vi "Get Or Create Cal Standard.vi"(11 "error in (no error)":errorcluster) -> (4 "Cal Standard Base out":refnum<class "Cal Standard Base.lvclass">, 15 "error out":errorcluster)   [LabVIEW 2023, in "RFFixtureCharact.Instruments.lvlib" / "Cal Standard Factory.lvclass"]
uses:
  Cal Standard Factory.lvclass
  Cal Standard Base/Cal Standard Base.lvclass
  Cal Standard Sim/Cal Standard Sim.lvclass
  C:/srd-semi-rfcal-software/AuxTools/STSRFFixtureCharactUtility/Source/Code Modules/Fixture/Instruments/Cal Standard/Cal Standard Base/Cal Standard Base.lvclass
  Cal Standard Base/Cal Standard Base.lvclass/Cal Standard Base.ctl
  Cal Standard Base/Properties/Read Instrument Info.vi
  Common/RFCalAndFixtureCharact.Common.lvlib
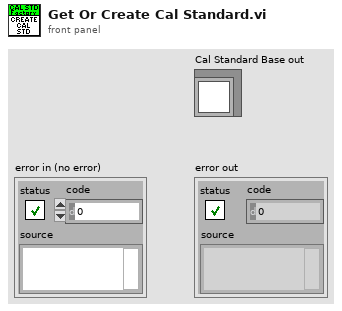
[diagram p1: front panel]
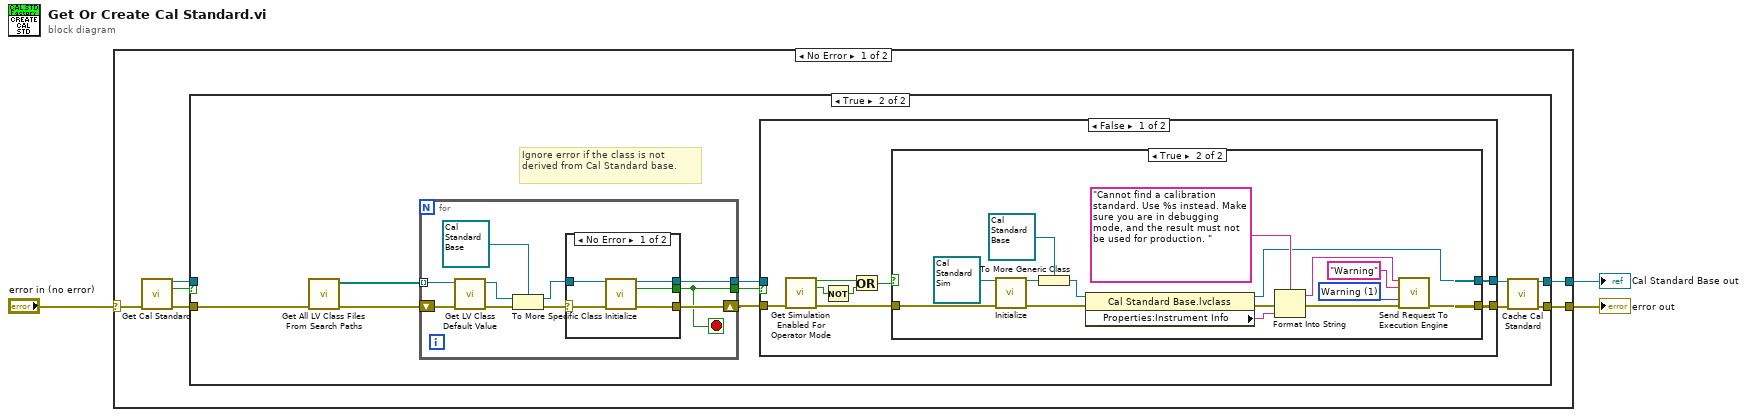
[diagram p0: block diagram]
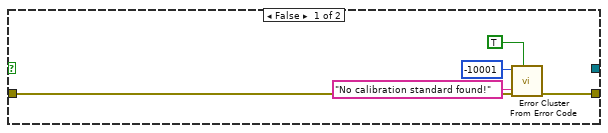
[diagram p3: hidden frame]
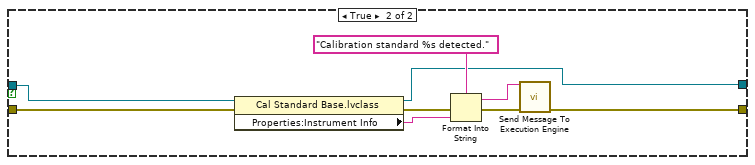
[diagram p4: hidden frame]
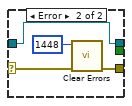
[diagram p5: hidden frame]
diagram:
  n1 = case shown="No Error" "error in (no error)" {
    selector: "error in (no error)" -> [w7 w78]
    tunnel: [w9 w78] -> w2
    tunnel: [w8 _] -> w1
    frame No Error {
      n2 = call "Get Cal Standard.vi"("error in (no error)"=w7) -> ("Cal Standard Base out"=w4:refnum<class "Cal Standard Base.lvclass">, "Not found"=w5:bool, "error out"=w6:errorcluster)  [unwired: 12 in]
      n3 = case shown="True" w5 {
        tunnel: [w11 w21] -> w9
        tunnel: [w10 w20] -> w8
        tunnel: w6 -> [w11 w13]
        tunnel: w4 -> [w10 _]
        frame False {
        }
        frame True {
          # "Ignore error if the class is not derived from Cal Standard base."
          n4 = call "Get All LV Class Files From Search Paths.vi"("error in"=w13) -> ("All Files in Dir"=w14:path[], "error out"=w12:errorcluster)  [unwired: 13 in]
          n5 = for {
            tunnel: [w68] -> w19
            shift-right: [w67] -> w18
            shift-left: w12 -> [w66]
            tunnel: w14 -> [w64] mode=indexing
            tunnel: [w59] -> w15
            stop <- w59 stop-if-true
            n6 = call <vilib>:"Get LV Class Default Value.vi"("error in (no error)"=w66, "class path"=w64) -> ("error out"=w65:errorcluster, "object"=w63:refnum<class>)  [unwired: 8 in]
            n7 = To More Specific Class(target class=refnum<class "Cal Standard Base.lvclass"> refnum ("STS Vector Fixture Charact.lvlib:Cal Standard Base.lvclass"), reference=w63, error in=w65) -> (specific class reference=w62:refnum<class "Cal Standard Base.lvclass">, error out=w61:errorcluster)
            n8 = case shown="No Error" w61 {
              selector: w61 -> [w72 w76]
              tunnel: [w71 w75] -> w68
              tunnel: [w70 w74] -> w67
              tunnel: w62 -> [w73 w75]
              tunnel: [w69 _] -> w59
              frame No Error {
                n9 = call-dynamic "Initialize.vi"("Cal Standard Base in"=w73, "error in (no error)"=w72) -> ("Cal Standard Base out"=w71:refnum<class "Cal Standard Base.lvclass">, "Found"=w69:bool, "error out"=w70:errorcluster)  [unwired: 11 in]
              }
              frame Error {
                n10 = call <vilib>:"Clear Errors.vi"("error in (no error)"=w76, "specific error code to clear (0: all)"=1448) -> ("error out"=w74:errorcluster)  [unwired: 4 in, 1 out]
              }
            }
          }
          n11 = case shown="False" w15 {
            tunnel: w18 -> [w29 w52]
            tunnel: w19 -> [_ w53]
            tunnel: [w27 w50] -> w16
            tunnel: [w28 w51] -> w17
            frame False {
              n12 = call "Get Simulation Enabled For Operator Mode.vi"("error in (no error)"=w29) -> ("Use Simulated Instrument?"=w24:bool, "Use Operator Mode?"=w22:bool, "error out"=w26:errorcluster)  [unwired: 12 in]
              n13 = Not(x=w22) -> (.not. x?=w23:bool)
              n14 = Or(x=w24, y=w23) -> (x .or. y?=w25:bool)
              n15 = case shown="True" w25 {
                tunnel: [w33 w38] -> w28
                tunnel: [_ w37] -> w27
                tunnel: w26 -> [w34 w35]
                frame False {
                  n16 = call <vilib>:"Error Cluster From Error Code.vi"("show call chain? (False)"=TRUE, "error in (no error)"=w34, "error message (\"\")"="No calibration standard found!" ("error message (\"\")"), "error code (0)"=-10001) -> ("error out"=w33:errorcluster)  [unwired: 5 in]
                }
                frame True {
                  w41 = 1 items=["Info", "Warning", "Error", "Action"] ("RequestContentType")
                  n17 = call-dynamic "Initialize.vi"("Cal Standard Sim in"=refnum<class "Cal Standard Sim.lvclass"> refnum ("STS Vector Fixture Charact.lvlib:Cal Standard Sim.lvclass"), "error in (no error)"=w35) -> ("Cal Standard Sim out"=w49:refnum<class "Cal Standard Sim.lvclass">, "error out"=w46:errorcluster)  [unwired: 11 in, 1 out]
                  n18 = To More Generic Class(target class=refnum<class "Cal Standard Base.lvclass"> refnum ("STS Vector Fixture Charact.lvlib:Cal Standard Base.lvclass"), reference=w49) -> (generic class reference=w45:refnum<class "Cal Standard Base.lvclass">)
                  n19 = property class="Cal Standard Base.lvclass"(reference=w45, error in=w46) -> (reference out=w37:refnum<class "Cal Standard Base.lvclass">, error out=w44:errorcluster, "Properties:Instrument Info"=w43:string)
                  n20 = Format Into String(format string="Cannot find a calibration standard. Use %s instead. Make sure you are in debugging mode, and the result must not be used for production. " ("message"), error in=w44, w43) -> (resulting string=w36:string, error out=w39:errorcluster)  [unwired: 1 in]
                  n21 = call "Send Request To Execution Engine.vi"("Request Message"=w36, "Request Header"="Warning" ("headerText"), "Request Content Type"=w41, "error in (no error)"=w39) -> ("error out"=w38:errorcluster)  [unwired: 10 in, 1 out]
                }
              }
            }
            frame True {
              n22 = property class="Cal Standard Base.lvclass"(reference=w53, error in=w52) -> (reference out=w50:refnum<class "Cal Standard Base.lvclass">, error out=w58:errorcluster, "Properties:Instrument Info"=w55:string)
              n23 = Format Into String(format string="Calibration standard %s detected.", error in=w58, w55) -> (resulting string=w54:string, error out=w57:errorcluster)  [unwired: 1 in]
              n24 = call "Send Message To Execution Engine.vi"("Message"=w54, "error in (no error)"=w57) -> ("error out"=w51:errorcluster)  [unwired: 13 in]
            }
          }
          n25 = call "Cache Cal Standard.vi"("Cal Standard Base in"=w16, "error in (no error)"=w17) -> ("Cal Standard Base out"=w20:refnum<class "Cal Standard Base.lvclass">, "error out"=w21:errorcluster)  [unwired: 12 in]
        }
      }
    }
    frame Error {
    }
  }
  "error out" <- w2
  "Cal Standard Base out" <- w1
